vi "索引数组.vi"() -> ()   [LabVIEW 2010]
panel:
  out "1页2行":dbl[](array[numeric]) format="%.2f"
  out "2列":dbl[](array[numeric]) format="%.2f"
  out "1页":dbl[][](array[numeric]) format="%.2f"
  out "1行2列":dbl format="%.2f"
  out "3行":dbl[](array[numeric]) format="%.2f"
  out "数组元素4":i32
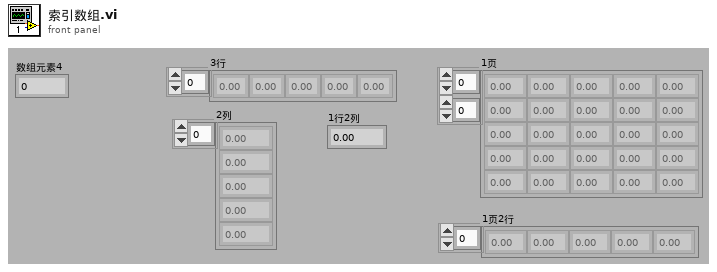
[diagram p1: front panel]
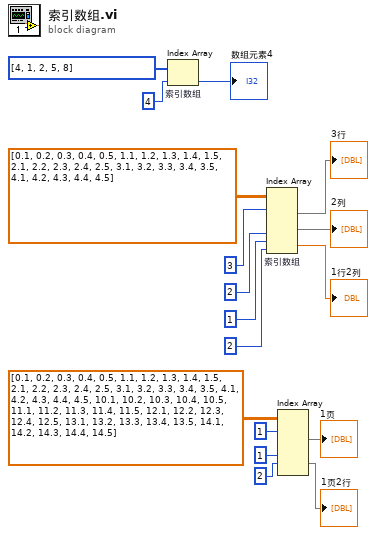
[diagram p0: block diagram]
diagram:
  n1 = Index Array "索引数组"(array=i32[] [4, 1, 2, 5, 8], index=4) -> (element=→"数组元素4":i32)
  n2 = Index Array "索引数组"(array=dbl[][] [[0.1, 0.2, 0.3, 0.4, 0.5], [1.1, 1.2, 1.3, 1.4, 1.5], [2.1, 2.2, 2.3, 2.4, 2.5], [3.1, 3.2, 3.3, 3.4, 3.5], [4.1, 4.2, 4.3, 4.4, 4.5]], index (row) #1=3 ("index"), index (col) #2=2, index (row) #3=1, index (col) #3=2) -> (element #1=→"3行":dbl[], element #2=→"2列":dbl[], element #3=→"1行2列":dbl)  [unwired: 2 in]
  n3 = Index Array(array=dbl[][][] [[[0.1, 0.2, 0.3, 0.4, 0.5], [1.1, 1.2, 1.3, 1.4, 1.5], [2.1, 2.2, 2.3, 2.4, 2.5], [3.1, 3.2, 3.3, 3.4, 3.5], [4.1, 4.2, 4.3, 4.4, 4.5]], [[10.1, 10.2, 10.3, 10.4, 10.5], [11.1, 11.2, 11.3, 11.4, 11.5], [12.1, 12.2, 12.3, 12.4, 12.5], [13.1, 13.2, 13.3, 13.4, 13.5], [14.1, 14.2, 14.3, 14.4, 14.5]]], index (dim 0) #1=1 ("index"), index (dim 0) #2=1, index (dim 1) #2=2) -> (element #1=→"1页":dbl[][], element #2=→"1页2行":dbl[])  [unwired: 3 in]
